vi "Actor Receive.vi"(11 "Actor in":refnum<class "Actor.lvclass">) -> (0 "error out":errorcluster, 2 "Msg":refnum<class "Msg Strategy.lvclass">, 3 "Actor out":refnum<class "Actor.lvclass">)   [LabVIEW 2021, in "jettl.lvlib" / "Actor.lvclass"]
uses:
  Actor.lvclass
  Msg Strategy/Msg Strategy.lvclass
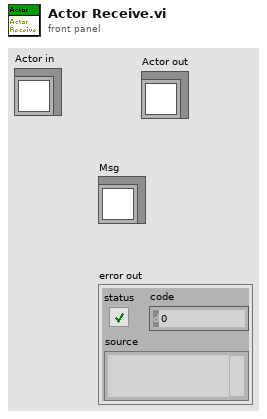
[diagram p1: front panel]
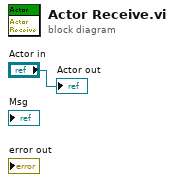
[diagram p0: block diagram]
diagram:
  "Actor out" <- "Actor in"
